vi "pmu_Check PMU Parameter Error.vi"(8 "error in (no error)":errorcluster, 10 "number of PMUs":u16=1, 11 "time base":u32=10000000) -> (0 "error out":errorcluster)   [LabVIEW 2011, in "NI_EP_PMU.lvlib"]
uses:
  <vilib>/addons/Electrical Power/PMU/NI_EP_PMU.lvlib
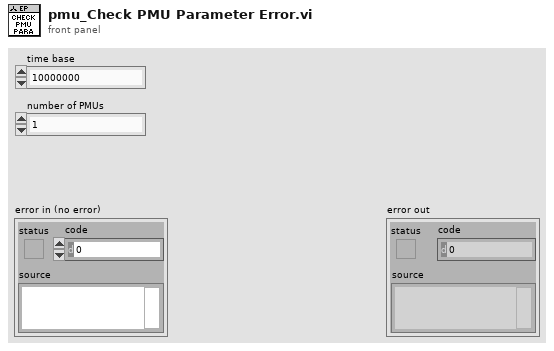
[diagram p1: front panel]
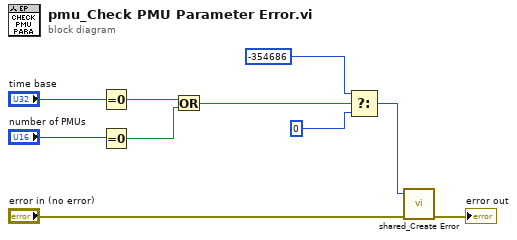
[diagram p0: block diagram]
diagram:
  n1 = Equal To 0?(x="time base") -> (x = 0?=w7:bool)
  n2 = Equal To 0?(x="number of PMUs") -> (x = 0?=w8:bool)
  n3 = Or(x=w7, y=w8) -> (x .or. y?=w6:bool)
  n4 = Select(t=-354686 ("error code (0)"), s=w6, f=0 ("error code (0)")) -> (s? t:f=w1:i32)
  n5 = call <vilib>:"shared_Create Error.vi"("error in (no error)"="error in (no error)", "error code (0)"=w1) -> ("error out"=→"error out":errorcluster)  [unwired: 9 in]
